vi "Set_Speed.vi"(5 "Channel Name (Calib Tweak)":string, 6 "Calib Tweak":dbl format="%.2f", 7 "Client Name":string, 8 "Channel Name (Volts/Amps)":string, 9 "Demanded Velocity":dbl format="%.2f", 10 "Channel Name (Velocity)":string) -> ()   [LabVIEW 2010]
uses:
  ADAM Client/Sub VIs/ADAM Controls/Update_scan_value.ctl
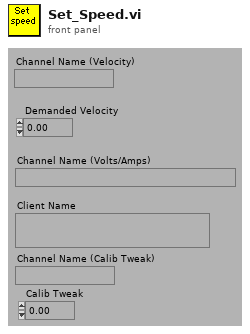
[diagram p1: front panel]
types:
  T1 = enum16{"Append to Global", "Read Global then Clear"}
  T2 = typedef "Update_scan_value.ctl" = cluster{"Channel Name":string, "New Value":dbl}
  T3 = typedef "Ch_description_ADAM.ctl" = cluster{"Ch Name":string, "Type":T4, "Function":T5, "Ch State":T6, "Calibration type":T7, "A":dbl, "B":dbl, "C":dbl, "D":dbl, "Comments":string, "Address":T8, "String":string, "Duty":u16}
  T4 = typedef "Module_type_ADAM.ctl" = enum16{"4011", "4012", "4013", "4014", "4016", "4017", "4018", "4021", "4050", "4052", "4053", "4060", "4080", "5000", "5017", "5018", "5024", "5051", "5056", "5060", "6060", "Tracker", "WEST", "GILL", "JEM", "VICI", "Vaisala", "DRUCK", "Run VI Named:", "IR2100", "PPT", "Comparator", "VIRTUAL", "Hold Value", "Read A", "Read Ch", "Coded", "Client Info", "Web Client", "X10", "Test"}
  T5 = typedef "Function_ADAM.ctl" = enum16{"Analogue Input", "Digital Input", "Event counter", "Event rate", "Analogue Output", "Digital Output", "Relay Output"}
  T6 = typedef "Channel_State.ctl" = enum16{"On", "Off", "Always On", "Always Off"}
  T7 = typedef "Calib_type_ADAM.ctl" = enum16{"Raw", "Bx + A", "Cx^2 + Bx + A", "Dx^3 + Cx^2 + Bx + A", "In Band", "Hi-Tec Q", "Hi-Tec M_dot", "Text"}
  T8 = typedef "Address.ctl" = cluster{"Main":i32, "Ch.":i32, "Sub":i32, "Port Name":string}
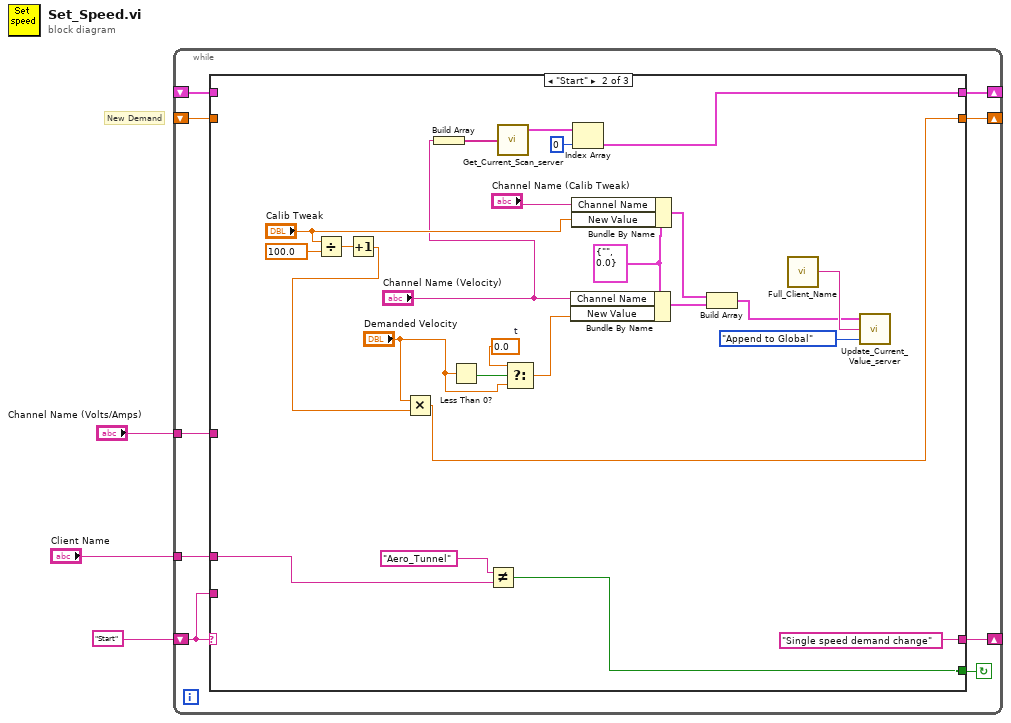
[diagram p0: block diagram]
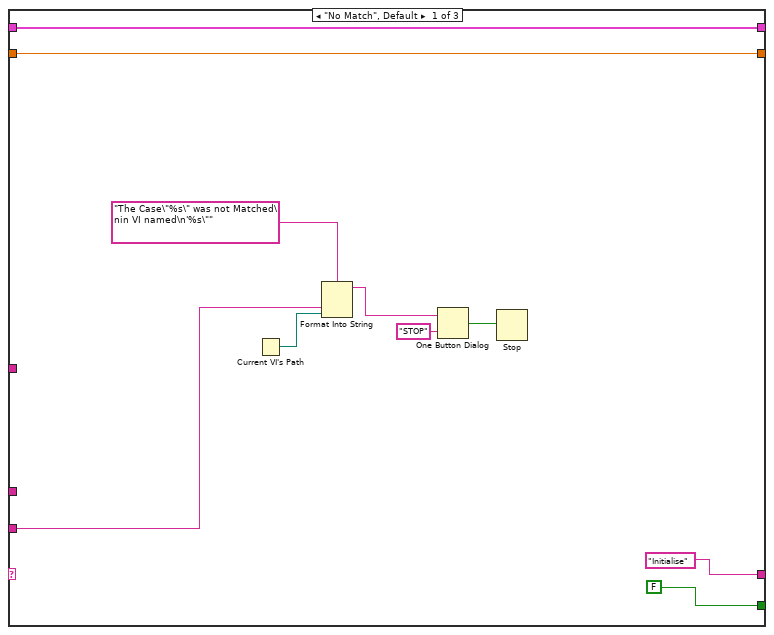
[diagram p2: hidden frame]
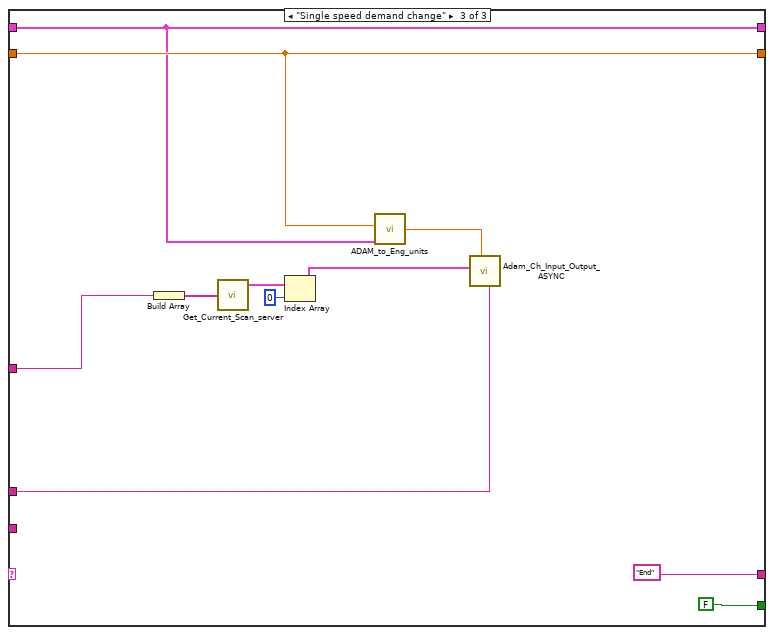
[diagram p3: hidden frame]
diagram:
  # "New Demand"
  n1 = while {
    shift-left: "Start" -> [w10]
    shift-right: [w11] -> _
    shift-right: [w7] -> _
    shift-left: _ -> [w8]
    tunnel: "Channel Name (Volts/Amps)" -> [w9]
    tunnel: "Client Name" -> [w6]
    shift-right: [w5] -> _
    shift-left: _ -> [w4]
    stop <- w12 continue-if-true
    n2 = case shown="\"Start\"" w10 {
      tunnel: [FALSE w23 FALSE] -> w12
      tunnel: ["Initialise" "Single speed demand change" "End"] -> w11
      tunnel: w10 -> [w17 _ _]
      tunnel: w9 -> [_ _ w53]
      tunnel: w8 -> [w14 _ w50]
      tunnel: [w14 w32 w50] -> w7
      tunnel: w6 -> [_ w24 w52]
      tunnel: [w13 w27 w48] -> w5
      tunnel: w4 -> [w13 _ w48]
      frame "No Match", Default {
        n3 = Current VI's Path() -> (path=w16:path)
        n4 = Format Into String(format string="The Case\"%s\" was not Matched\nin VI named\n'%s\"" ("Format String"), w17, w16) -> (resulting string=w20:string)  [unwired: 2 in, 1 out]
        n5 = One Button Dialog(message=w20, button name ("OK")="STOP") -> (true=w18:bool)
        n6 = Stop(stop? (T)=w18) -> ()
      }
      frame "Start" {
        w38 = T2 {"Channel Name"="", "New Value"=0.0} ("Update Scan Value Cluster")
        w44 = 0.0  # t
        n7 = Divide(x="Calib Tweak", y=100.0) -> (x/y=w43:dbl)
        n8 = Increment(x=w43) -> (x+1=w46:dbl)
        n9 = Multiply(x="Demanded Velocity", y=w46) -> (x*y=w32:dbl)
        n10 = Build Array("Channel Name (Velocity)") -> (w31:string[])
        n11 = Less Than 0?(x="Demanded Velocity") -> (x < 0?=w36:bool)
        n12 = Not Equal?(x="Aero_Tunnel", y=w24) -> (x != y?=w23:bool)
        n13 = call "Get_Current_Scan_server.vi"("Desired Channels"=w31) -> ("Ch Description Array"=w28:T3[])  [unwired: 2 out]
        n14 = Select(t=w44, s=w36, f="Demanded Velocity") -> (s? t:f=w45:dbl)
        n15 = Bundle By Name(cluster=w38, "Channel Name"="Channel Name (Velocity)", "New Value"=w45) -> (w34:T2)
        n16 = Bundle By Name(cluster=w38, "Channel Name"="Channel Name (Calib Tweak)", "New Value"="Calib Tweak") -> (w40:T2)
        n17 = Index Array(array=w28, index=0) -> (element=w27:T3)
        n18 = Build Array(w40, w34) -> (w35:T2[])
        n19 = call "Full_Client_Name.vi"() -> ("Client Name"=w37:string)
        n20 = call "Update_Current_Value_server.vi"("Mode"=T1."Append to Global", "Client HD name"=w37, "Update array in"=w35) -> ()  [unwired: 1 out]
      }
      frame "Single speed demand change" {
        n21 = Build Array(w53) -> (w56:string[])
        n22 = call "Get_Current_Scan_server.vi"("Desired Channels"=w56) -> ("Ch Description Array"=w54:T3[])  [unwired: 2 out]
        n23 = Index Array(array=w54, index=0 ("Index")) -> (element=w51:T3)
        n24 = call "ADAM_to_Eng_units.vi"("Ch Description"=w48, "Raw"=w50) -> ("Calibrated units"=w49:dbl)  [unwired: 4 out]
        n25 = call "Adam_Ch_Input_Output_ASYNC.vi"("Client Name"=w52, "Value to Output"=w49, "Ch Discription"=w51) -> ()  [unwired: 4 in, 5 out]
      }
    }
  }
